vi "Query Registry.vi"(6 "use Regex? (F)":bool, 8 "error in (no error)":errorcluster, 9 "Search string":string=".*", 10 "Search Key (FQN)":T1, 11 "Registry in":refnum<data-value>) -> (0 "error out":errorcluster, 1 "Nodes":refnum<class "UniqueName.lvclass">[](array[class]), 2 "Node":refnum<class "UniqueName.lvclass">, 3 "Registry":refnum<data-value>, 4 "found?":bool)   [LabVIEW 2013, in "UniqueName.lvlib" / "NameRegistry.lvclass"]
uses:
  NameRegistry.lvclass
  UniqueNameClass/Key.ctl
  UniqueNameClass/UniqueName.lvclass
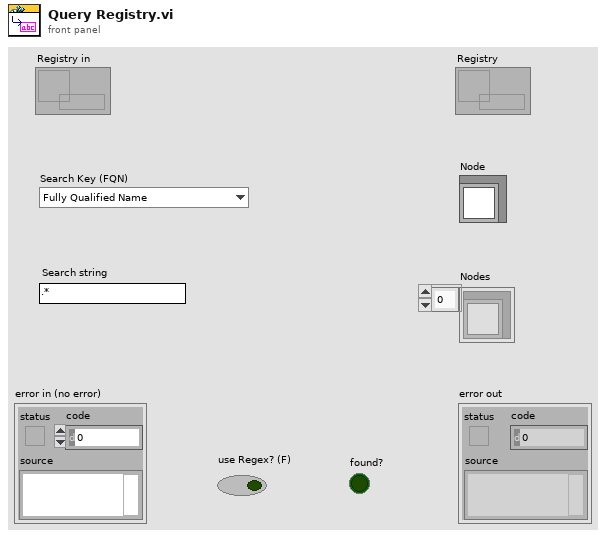
[diagram p1: front panel]
types:
  T1 = typedef "UniqueName.lvlib/UniqueName.lvclass/Key.ctl" = enum16{"Fully Qualified Name", "Unique Name", "Given Name", "Parent Fully Qualified Name", "UUID"}
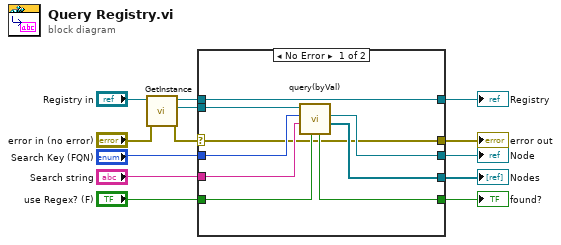
[diagram p0: block diagram]
diagram:
  n1 = call "GetInstance.vi"("error in (no error)"="error in (no error)", "Registry in"="Registry in") -> ("error out"=w1:errorcluster, "Instance"=w3:refnum<class "NameRegistry.lvclass">, "Registry out"=w4:refnum<data-value>)  [unwired: 7 in]
  n2 = case shown="No Error" w1 {
    selector: w1 -> [w14 w23]
    tunnel: w4 -> [w16 w24]
    tunnel: [w16 w24] -> w13
    tunnel: [w14 w23] -> w12
    tunnel: "use Regex? (F)" -> [w20 _]
    tunnel: "Search string" -> [w21 _]
    tunnel: "Search Key (FQN)" -> [w22 _]
    tunnel: [w18 _] -> w8
    tunnel: [w19 _] -> w7
    tunnel: [w17 _] -> w6
    tunnel: w3 -> [w15 _]
    frame No Error {
      n3 = call "query(byVal).vi"("use Regex? (F)"=w20, "Search string"=w21, "Search Key (FQN)"=w22, "Instance"=w15) -> ("Nodes"=w18:refnum<class "UniqueName.lvclass">[], "First Node"=w19:refnum<class "UniqueName.lvclass">, "found?"=w17:bool)  [unwired: 4 in, 1 out]
    }
    frame Error {
    }
  }
  "error out" <- w12
  "Registry" <- w13
  "Node" <- w7
  "Nodes" <- w8
  "found?" <- w6
